vi "track_particles_2d.vi"(4 "Output to Image":bool=TRUE, 5 "margin":i32=15, 6 "Method":T2(ring), 7 "ROIs":i32[][](array[numeric]), 9 "Threshold":sgl(slide)=128.0 scale=0.0..255.0, 11 "Image Src":T1) -> (2 "Positions":cluster{dbl, dbl}[](array[cluster]), 3 "Image Out":T1)   [LabVIEW 2010]
uses:
  <vilib>/vision/Image Controls.llb/IMAQ Image.ctl
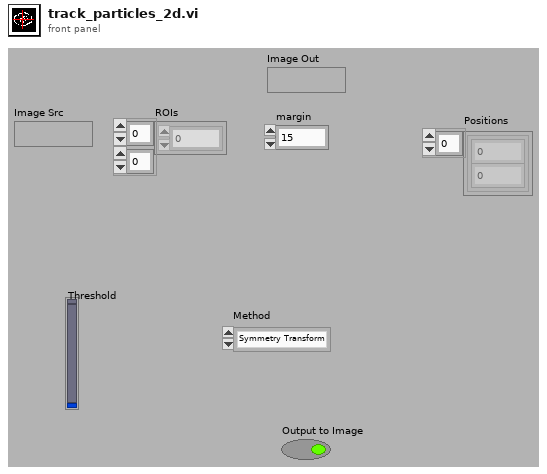
[diagram p1: front panel]
types:
  T1 = typedef "IMAQ Image.ctl" = refnum<image>
  T2 = enum16{"Symmetry Transform", "Centre of Mass", "CoM plus line information", "Inverted CoM"}
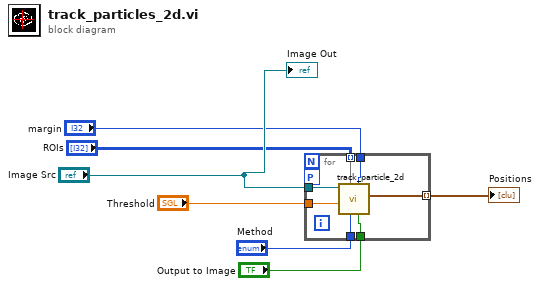
[diagram p0: block diagram]
diagram:
  n1 = for {
    tunnel: "Image Src" -> [w14]
    tunnel: "ROIs" -> [w13] mode=indexing
    tunnel: "Threshold" -> [w12]
    tunnel: "Method" -> [w11]
    tunnel: "Output to Image" -> [w10]
    tunnel: "margin" -> [w9]
    tunnel: [w8] -> w1 mode=indexing
    workers-P: _ -> [_]
    n2 = call "track_particle_2d.vi"("Output to Image"=w10, "margin"=w9, "Method"=w11, "Optional Rectangle"=w13, "Threshold"=w12, "Image Src"=w14) -> ("Particle Position"=w8:cluster{dbl, dbl})  [unwired: 3 in, 2 out]
  }
  "Positions" <- w1
  "Image Out" <- "Image Src"
